vi "SR830_Open.vi"(8 "Error In":errorcluster caption="错误输入", 10 "Sample Rate (0: 62.5 mHz)":u16(ring)=11 items=["62.5 mHz", "125 mHz", "250 mHz", "500 mHz", "1 Hz", "2 Hz", "4 Hz", "8Hz", "16 Hz", "32 Hz", "64 Hz", "128 Hz", "256 Hz", "512 Hz", "Trigger "], 11 "VISA 输入":refnum<visa-resource-name>="GPIB0::7::INSTR") -> (0 "Error Out":errorcluster caption="错误输出")   [LabVIEW 2020]
uses:
  lib/SR830/SR830.lvlib
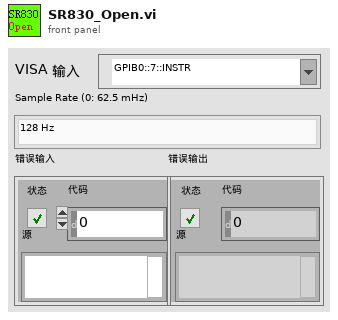
[diagram p1: front panel]
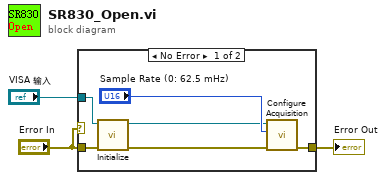
[diagram p0: block diagram]
diagram:
  n1 = case shown="No Error" "Error In" {
    tunnel: "Error In" -> [w8 w10]
    tunnel: "VISA 输入" -> [w9 _]
    tunnel: [w4 w10] -> w1
    frame No Error {
      n2 = call "Initialize.vi"("error in (no error)"=w8, "VISA resource name"=w9) -> ("error out"=w5:errorcluster, "VISA resource name out"=w6:refnum<visa-resource-name>)  [unwired: 8 in]
      n3 = call "Configure Acquisition.vi"("error in (no error)"=w5, "Sample Rate (0: 62.5 mHz)"="Sample Rate (0: 62.5 mHz)", "VISA resource name"=w6) -> ("error out"=w4:errorcluster)  [unwired: 7 in, 1 out]
    }
    frame Error {
    }
  }
  "Error Out" <- w1
